vi "Mass Memory.vi"(8 "error in (no error)":errorcluster, 9 "Record Number (0)":i16 min=0 max=19 step=1, 10 "Mode (Load:T)":bool=TRUE, 11 "VISA resource name":refnum<visa-resource-name>) -> (0 "error out":errorcluster, 3 "VISA resource name out":refnum<visa-resource-name>)   [LabVIEW 2015, in "Agilent 428X Series.lvlib"]
doc: "The Mass Memory function loads or stores setting data from/to the internal EEPROM and the external memory card."
uses:
  Agilent 428X Series.lvlib
panel:
  # "Load\nStore"
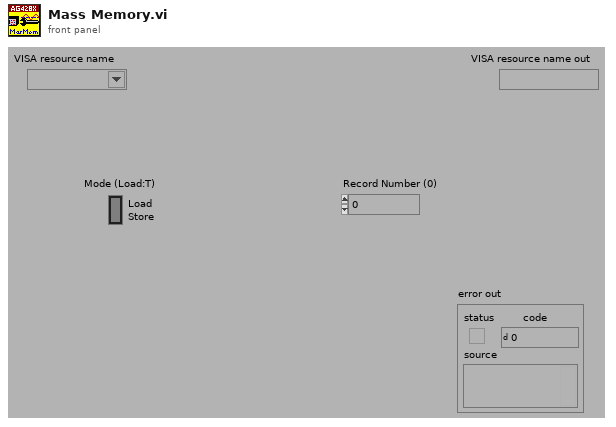
[diagram p1: front panel]
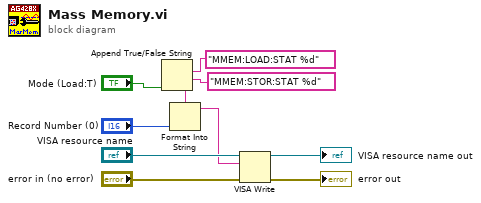
[diagram p0: block diagram]
diagram:
  n1 = Append True/False String(1:"Mode (Load:T)", 2:"MMEM:STOR:STAT %d", 3:"MMEM:LOAD:STAT %d") -> (0:w3:string)  [unwired: 1 in]
  n2 = Format Into String(format string=w3, "Record Number (0)") -> (resulting string=w1:string)  [unwired: 2 in, 1 out]
  n3 = VISA Write(VISA resource name="VISA resource name", write buffer=w1, error in (no error)="error in (no error)") -> (VISA resource name out=→"VISA resource name out":refnum<visa-resource-name>, error out=→"error out":errorcluster)  [unwired: 1 out]
